vi "From JSON.vi"(8 "error in (no error)":errorcluster, 11 "JSON":string) -> (0 "error out":errorcluster, 3 "Version":refnum<class "Version.lvclass">)   [LabVIEW 2020, in "GCentral-API.lvlib" / "Version.lvclass"]
uses:
  Version.lvclass
  Repo Type.ctl
  Version.lvclass/Version.ctl
  gpm_packages/@mgi/semver/Semver/Semver.lvclass
  GCentral-API.lvlib
  neg-pkg/JSON/JSON.lvlib
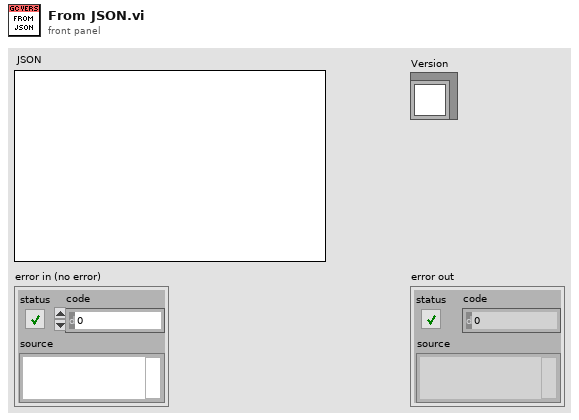
[diagram p1: front panel]
types:
  T1 = typedef "GCentral-API.lvlib/Repo Type.ctl" = enum16{"VIPM", "GPM", "NIPM"}
  T2 = typedef "JSON.lvlib/JSON Item Type.ctl" = enum16{"unknown", "null", "Array", "Object", "String", "Number", "Boolean"}
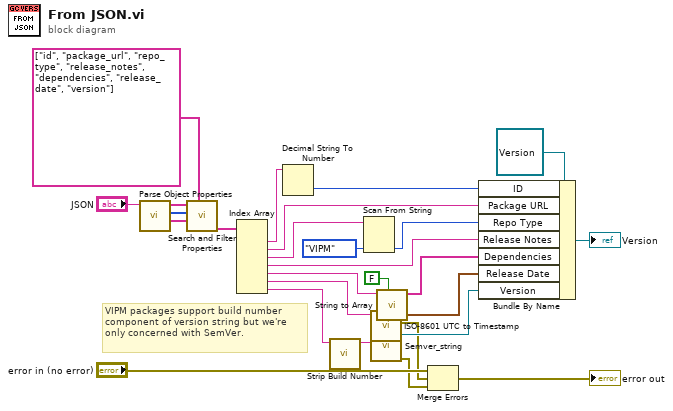
[diagram p0: block diagram]
diagram:
  # "VIPM packages support build number component of version string but we're only concerned with SemVer."
  n1 = call "Parse Object Properties.vi"("JSON String"="JSON") -> ("Values"=w14:string[], "Item Types"=w15:T2[], "Keys"=w16:string[])  [unwired: 7 in, 1 out]
  n2 = call "Search and Filter Properties.vi"("Search Keys"=string[] ["id", "package_url", "repo_type", "release_notes", "dependencies", "release_date", "version"], "Values In"=w14, "Types In"=w15, "Keys In"=w16) -> ("Filtered Values"=w12:string[])  [unwired: 2 in, 5 out]
  n3 = Index Array(array=w12) -> (element #1=w11:string, element #2=w9:string, element #3=w8:string, element #4=w7:string, element #5=w6:string, element #6=w3:string, element #7=w1:string)  [unwired: 7 in]
  n4 = Decimal String To Number(string=w11) -> (number=w10:i32)  [unwired: 2 in, 1 out]
  n5 = call "Strip Build Number.vi"("Version String In"=w1) -> ("Version String"=w2:string)  [unwired: 10 in]
  n6 = Scan From String(input string=w8, default 1=Repo_Type."VIPM" ("Repo Type")) -> (output 1=w25:T1)  [unwired: 3 in, 3 out]
  n7 = call "ISO-8601 UTC to Timestamp.vi"("ISO-8601"=w3) -> ("error out"=w19:errorcluster, "time stamp"=w22:timestamp)  [unwired: 9 in]
  n8 = call "Semver_string.vi"("Version"=w2) -> ("error out"=w20:errorcluster, "Semver out"=w26:refnum<class "Semver.lvclass">)  [unwired: 9 in]
  n9 = call "String to Array.vi"("Quoted Strings? (F)"=FALSE, "Array String In"=w6) -> ("JSON Strings"=w4:string[])  [unwired: 9 in]
  n10 = Merge Errors("error in (no error)", w19, w20) -> (→"error out":errorcluster)
  n11 = Bundle By Name(cluster=refnum<class "Version.lvclass"> refnum ("GCentral-API.lvlib:Version.lvclass"), "ID"=w10, "Package URL"=w9, "Repo Type"=w25, "Release Notes"=w7, "Dependencies"=w4, "Release Date"=w22, "Version"=w26) -> (→"Version":refnum<class "Version.lvclass">)
